vi "LEBITVacuum.WriteToFile.vi"(0 "convert eol? (no:F)":bool, 3 "append to file? (new file:F)":bool, 4 "character string":string, 5 "file path (dialog if empty)":path) -> (2 "new file path (Not A Path if cancelled)":path)   [LabVIEW 2014, in "LEBITVacuum.lvlib"]
doc: "Writes a <B>character string</B> to a new byte stream file or appends the string to an existing file. The VI opens or creates the file before writing to it and closes it afterwards."
uses:
  LEBITVacuum.lvlib
panel:
  in  "prompt":string="Choose file to write."
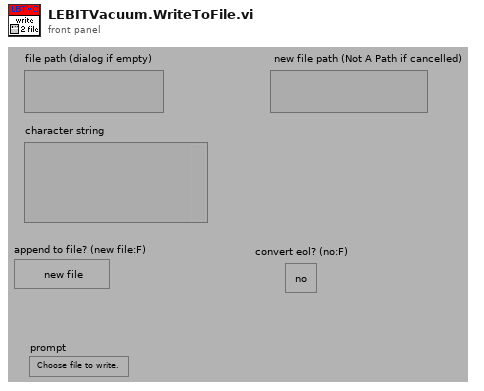
[diagram p1: front panel]
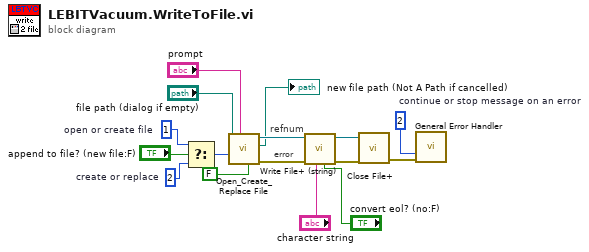
[diagram p0: block diagram]
diagram:
  w6 = i16 2  # create or replace
  w14 = 2  # continue or stop message on an error
  w9 = i16 1  # open or create file
  # "error"
  # "refnum"
  n1 = Select(t=w9, s="append to file? (new file:F)", f=w6) -> (s? t:f=w11:i16)
  n2 = call <vilib>:"Open_Create_Replace File.vi"("advisory dialog? (display:T)"=FALSE, "prompt"="prompt", "function (open:0)"=w11, "file path"="file path (dialog if empty)") -> ("error out"=w15:errorcluster, "new file path"=→"new file path (Not A Path if cancelled)":path, "refnum"=w5:refnum<file>)  [unwired: 4 in, 1 out]
  n3 = call <vilib>:"Write File+ (string).vi"("convert eol? (no:F)"="convert eol? (no:F)", "string"="character string", "error in (no error)"=w15, "refnum"=w5) -> ("error out"=w13:errorcluster, "dup refnum"=w12:refnum<file>)  [unwired: 3 in, 1 out]
  n4 = call <vilib>:"Close File+.vi"("error in (no error)"=w13, "refnum"=w12) -> ("error out"=w10:errorcluster)  [unwired: 3 in, 2 out]
  n5 = call <vilib>:"General Error Handler.vi"("type of dialog (OK msg:1)"=w14, "error in (no error)"=w10) -> ()  [unwired: 9 in, 5 out]
